vi "Get Errors.vi"(10 "Assertions":T1[](array[typedef])) -> (2 "Errors":T1[](array[typedef]))   [LabVIEW 2013, in "JUnit for Azure Pipelines.lvclass"]
uses:
  JUnit for Azure Pipelines.lvclass
  <vilib>/addons/_JKI Toolkits/Caraya/classes/Test Result/Assert Event Data (Extended).ctl
  <vilib>/addons/_JKI Toolkits/Caraya/classes/Test Result/Test Result.lvclass
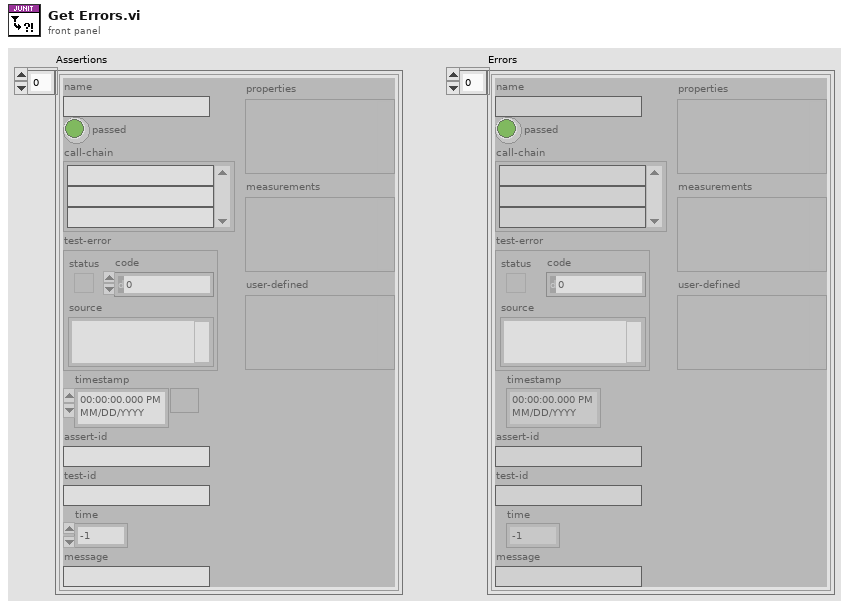
[diagram p1: front panel]
types:
  T1 = typedef "Caraya.lvlib/Test Result.lvclass/Assert Event Data (Extended).ctl" = cluster{"name":string, "passed":bool, "call-chain":string[], "test-error":errorcluster, "timestamp":timestamp, "assert-id":string, "test-id":string, "time":dbl, "message":string, "properties":variant, "measurements":variant, "user-defined":variant}
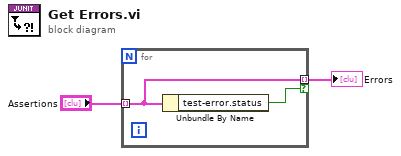
[diagram p0: block diagram]
diagram:
  n1 = for {
    tunnel: "Assertions" -> [w4] mode=indexing
    tunnel: [w4] -> w1 mode=indexing if=w3
    n2 = Unbundle By Name(w4) -> ("test-error.status"=w3:bool)
  }
  "Errors" <- w1
